vi "SetInbitTrigger.vi"(8 "error in (no error)":errorcluster, 10 "Inbit array":bool[](array[boolean])=[TRUE, FALSE, FALSE, FALSE, FALSE, FALSE, FALSE, FALSE, FALSE, FALSE, FALSE, FALSE, FALSE, FALSE, FALSE, FALSE], 11 "Refnum in":refnum<k21>="Inbits") -> (0 "error out":errorcluster, 3 "Refnum out":refnum<k21>="Inbits")   [LabVIEW 2018]
uses:
  <resource>/objmgr/daqmx.rc
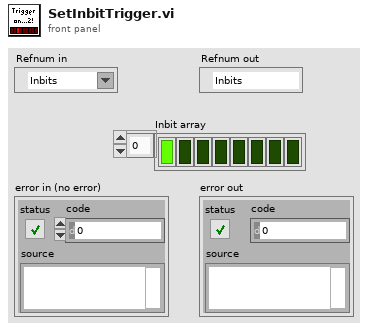
[diagram p1: front panel]
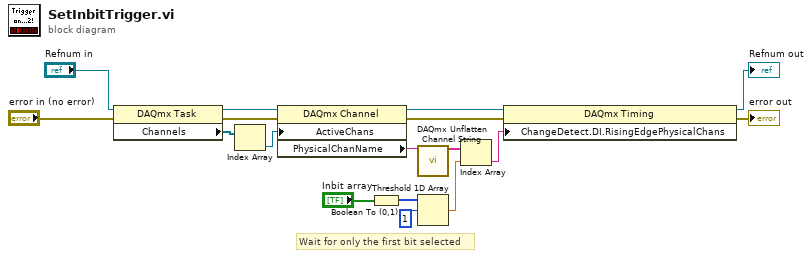
[diagram p0: block diagram]
diagram:
  # "Wait for only the first bit selected"
  n1 = property class="DAQmx Task"(reference="Refnum in", error in="error in (no error)") -> (reference out=w8:refnum<k21>, error out=w12:errorcluster, "Channels"=w9:refnum<k21>[])
  n2 = Index Array(array=w9) -> (element=w10:refnum<k21>)  [unwired: 1 in]
  n3 = property class="DAQmx Channel"(reference=w8, error in=w12, "ActiveChans"=w10) -> (reference out=w14:refnum<k21>, error out=w15:errorcluster, "PhysicalChanName"=w11:tag)
  n4 = Boolean To (0,1)(Boolean="Inbit array") -> (0, 1=w3:i16[])
  n5 = call <vilib>:"DAQmx Unflatten Channel String.vi"("names in"=w11) -> ("names out"=w16:string[])  [unwired: 13 in, 1 out]
  n6 = Threshold 1D Array(2:1, 3:w3) -> (0:w1:dbl)  [unwired: 1 in]
  n7 = Index Array(array=w16, index=w1) -> (element=w17:string)
  n8 = property class="DAQmx Timing"(reference=w14, error in=w15, "ChangeDetect.DI.RisingEdgePhysicalChans"=w17) -> (reference out=→"Refnum out":refnum<k21>, error out=→"error out":errorcluster)
